vi "getTemperature.vi"(6 "Channel":i32, 8 "error in (no error)":errorcluster, 11 "Inst.TC in":refnum<class "Inst.TC.lvclass">) -> (0 "error out":errorcluster, 1 "Status":string, 2 "Temperature (mK)":dbl, 3 "Inst.TC out":refnum<class "Inst.TC.lvclass">, 4 "Finished?":bool)   [LabVIEW 2019, in "Inst.TC.lvclass"]
uses:
  Inst.TC.lvclass
  <userlib>/LevyLab/Instrument Framework/Instrument Types/Cryostat/Instrument.Cryostat.lvclass
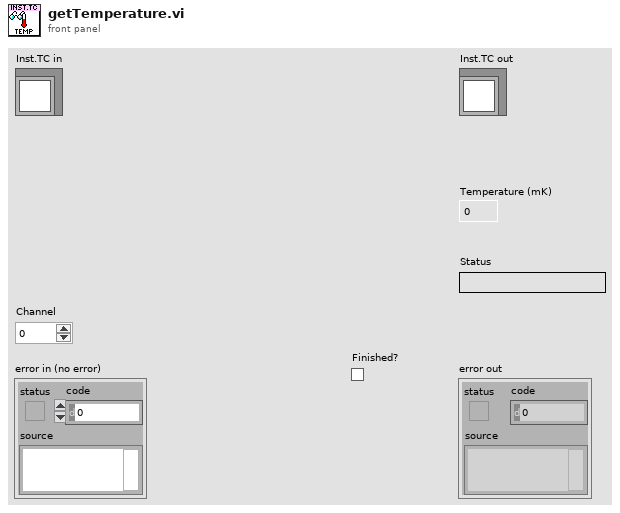
[diagram p1: front panel]
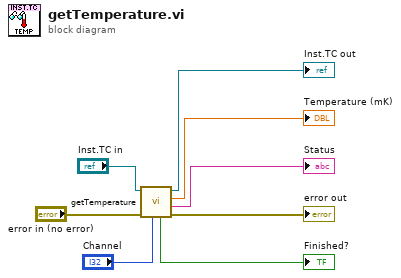
[diagram p0: block diagram]
diagram:
  n1 = call-parent "getTemperature.vi"("Channel"="Channel", "error in (no error)"="error in (no error)", "Instrument.Cryostat in"="Inst.TC in") -> ("error out"=→"error out":errorcluster, "Status"=→"Status":string, "Temperature (K)"=→"Temperature (mK)":dbl, "Instrument.Cryostat out"=→"Inst.TC out":refnum<class "Inst.TC.lvclass">, "Finished?"=→"Finished?":bool)  [unwired: 4 in]
